vi "MM9.InitDAC.vi"(0 "i ref in":refnum<vi>, 2 "InitObjs":string[](array[string]), 3 "ms timeout (10000)":i32=10000, 5 "error in (no error)":errorcluster) -> (14 "i ref out":refnum<vi>, 16 "InitObjs out":string[](array[string]), 17 "timed out":bool, 19 "error out":errorcluster)   [LabVIEW 2014, in "MM9.lvlib"]
doc: "Initializes the DAC that produces a two stage ramp when triggered."
uses:
  MM9.lvlib
  CS_Core/CSSystem/CoreDefs/CoreDefs.call_type.ctl
  CS_Core/BaseProcess/BaseProcess.descriptor string definition.ctl
  CS_Core/CSSystem/CoreDefs/CoreDefs.rawDataType.ctl
  CS_Core/CSSystem/CoreLib/CoreLib.int 2 byte array.vi
  CS_Core/BaseProcess/BaseProcess.lvlib
  LEBITLib/LEBITLib.lvlib
  CS_Core/CSSystem/CoreLib/CoreLib.lvlib
panel:
  in  "call cluster type":T1={"Object"="", "Selector"="", "CallType"=enum."synchronous", "Async Object"="", "Async Selector"="", "Data Descriptor"="", "Data"=[], "Error #"=0, "Expire"=0}
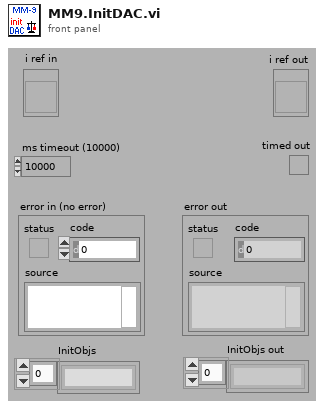
[diagram p1: front panel]
types:
  T1 = typedef "CoreDefs.call_type.ctl" = cluster{"Object":string, "Selector":string, "CallType":enum16{"simple", "synchronous", "asynchronous"}, "Async Object":string, "Async Selector":string, "Data Descriptor":T2, "Data":T3, "Error #":i32, "Expire":u32}
  T2 = typedef "BaseProcess.lvlib/BaseProcess.descriptor string definition.ctl" = string
  T3 = typedef "CoreDefs.rawDataType.ctl" = i8[]
  T4 = typedef "MM9.lvlib/MM9.i attribute.ctl" = cluster{"UsedObjs":string[], "ActScanStep":i32[], "AbortRequest":bool, "StopRequest":bool, "# cycles":i32, "Connected":bool, "MMStatus":T5, "# data":i32, "DIMServices":cluster{"MM6StatusString":string, "MM6StatusID":i32, "discArchiver":string, "discArchiverID":i32, "eventBuilder":string, "eventBuilderID":i32, "GUIIDString":string, "GUIIDStringID":i32}, "dataFile":string, "PGRunning":T6, "ConfigData":T7, "ExtraDataSets":T22}
  T5 = typedef "MM9.lvlib/MM9.status.ctl" = enum16{"loaded", "load_error", "config", "config_error", "init", "init_error", "data_reset", "data_reset_error", "running", "start_error", "run_error", "abort_requested", "aborted", "stop_requested", "stopped", "stop_error", "Connected", "NOTConnected"}
  T6 = typedef "PPG_ABC.lvlib/PPG_ABC.PG_Running.ctl" = i32
  T7 = typedef "LEBITDefs9.lvlib/LEBITDefs.ConfigData.ctl" = cluster{"GenConfig":T8, "Configs":T10[]}
  T8 = typedef "LEBITDefs9.lvlib/LEBITDefs.GenConfig.ctl" = cluster{"Mode":i32, "Logs":T9[]}
  T9 = typedef "LEBITDefs9.lvlib/LEBITDefs.Log.ctl" = cluster{"Name":string, "FctName":string, "Special":string}
  T10 = typedef "LEBITDefs9.lvlib/LEBITDefs.OneConfig.ctl" = cluster{"MCA":T11, "Timing":T12, "Scans":T15[], "FreqDevs":T16[], "CleanDev":T17, "NrCycles":i32, "Specials":T19[], "Delays":T20[], "DAC":T21}
  T11 = typedef "LEBITDefs9.lvlib/LEBITDefs.MCA.ctl" = cluster{"Name":string, "Address":string, "NrChannels":i32, "Gate":i32, "NrPipse":i32, "AcqDelay":i32}
  T12 = typedef "LEBITDefs9.lvlib/LEBITDefs.Timing.ctl" = cluster{"TimeTables":cluster{"TimeTable":T13}[], "Memories":T14[], "ScanX":string, "ScanY":string}
  T13 = typedef "LEBITDefs9.lvlib/LEBITDefs.Timetable.ctl" = dbl[]
  T14 = typedef "LEBITDefs9.lvlib/LEBITDefs.Memory.ctl" = cluster{"Device":string, "ExtTrig":bool, "TT2Use":i32, "PatternTable":string[]}
  T15 = typedef "LEBITDefs9.lvlib/LEBITDefs.ScanDev.ctl" = cluster{"Name":string, "FctName":string, "Values":dbl[], "NrScanVals":i32, "Special":string}
  T16 = typedef "LEBITDefs9.lvlib/LEBITDefs.FreqDev.ctl" = cluster{"Name":string, "Amp":dbl, "CenterFreq":dbl, "Time":dbl}
  T17 = typedef "LEBITDefs9.lvlib/LEBITDefs.CleanDev.ctl" = cluster{"Name":string, "CleanData":T18[]}
  T18 = typedef "LEBITDefs9.lvlib/LEBITDefs.CleanDataType.ctl" = cluster{"Amp":dbl, "Center":dbl, "Plus":dbl, "Minus":dbl, "Time":dbl}
  T19 = typedef "LEBITDefs9.lvlib/LEBITDefs.Special.ctl" = cluster{"Name":string, "FctName":string, "VerySpecial":string, "Data":dbl}
  T20 = typedef "LEBITDefs9.lvlib/LEBITDefs.Delay.ctl" = cluster{"Name":string, "Delay":dbl}
  T21 = typedef "LEBITDefs9.lvlib/LEBITDefs.DAC.ctl" = cluster{"Name":string, "Step1":i32, "Step2":i32}
  T22 = typedef "LEBITDefs9.lvlib/LEBITDefs.ExtraData.ctl" = cluster{"Ions":cluster{"ExcitIonMass":string, "ExcitIonCharge":i32, "CleanIons":cluster{"CleanIonMass":string, "CleanIonCharge":i32}[]}, "TimingDescription":cluster{"TimeTableDescription":cluster{"Times":string[]}[], "PatternTableDescription":cluster{"Pattern":string[]}[]}, "ScanUnits":string[]}[]
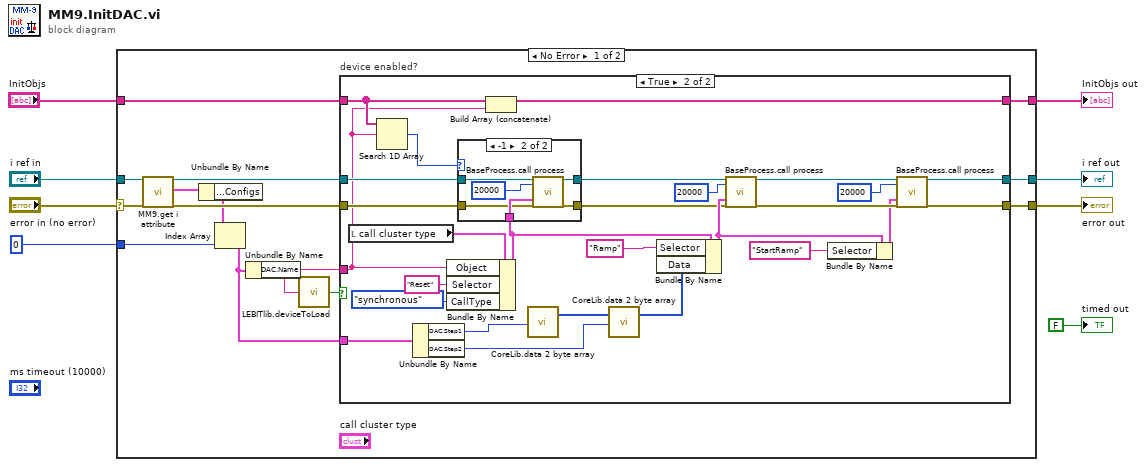
[diagram p0: block diagram]
diagram:
  n1 = case shown="No Error" "error in (no error)" {
    selector: "error in (no error)" -> [w15 w61]
    tunnel: "i ref in" -> [w22 w62]
    tunnel: [w20 w62] -> w7
    tunnel: [w19 w61] -> w6
    tunnel: "InitObjs" -> [w17 w63]
    tunnel: [w16 w63] -> w3
    tunnel: 0 ("index") -> [w9 _]
    frame No Error {
      n2 = call "MM9.get i attribute.vi"("i ref in"=w22, "error in (no error)"=w15) -> ("i ref out"=w21:refnum<vi>, "i attribute"=w11:T4, "error out"=w18:errorcluster)  [unwired: 15 in]
      n3 = Unbundle By Name(w11) -> ("ConfigData.Configs"=w12:T10[])
      n4 = Index Array(array=w12, index=w9) -> (element=w10:T10)
      n5 = Unbundle By Name(w10) -> ("DAC.Name"=w13:string)
      n6 = call "LEBITlib.deviceToLoad.vi"("DeviceName"=w13) -> ("DeviceIsToLoad"=w14:bool)
      n7 = case "device enabled?" shown="True" w14 {
        tunnel: [w25 w31] -> w20
        tunnel: [w24 w30] -> w19
        tunnel: w13 -> [_ w34]
        tunnel: w10 -> [_ w40]
        tunnel: w21 -> [w25 w39]
        tunnel: w18 -> [w24 w38]
        tunnel: w17 -> [w23 w35]
        tunnel: [w23 w33] -> w16
        frame False {
        }
        frame True {
          n8 = local read "call cluster type"() -> (w47:T1)
          n9 = Search 1D Array(1D array=w35, element=w34) -> (index of element=w36:i32)  [unwired: 1 in]
          n10 = Unbundle By Name(w40) -> ("DAC.Step1"=w27:i32, "DAC.Step2"=w26:i32)
          n11 = Bundle By Name(cluster=w47, "Object"=w34, "Selector"="Reset", "CallType"=enum16{"simple", "synchronous", "asynchronous"}."synchronous") -> (w48:T1)
          n12 = case shown="-1" w36 {
            tunnel: [w54 w59] -> w49
            tunnel: w48 -> [_ w58]
            tunnel: w39 -> [w54 w57]
            tunnel: w38 -> [w53 w56]
            tunnel: [w53 w55] -> w37
            frame 0, Default {
            }
            frame -1 {
              n13 = call "BaseProcess.call process.vi"("i ref in"=w57, "timeout (ms)"=20000, "call cluster in"=w58, "error in (no error)"=w56) -> ("i ref out"=w59:refnum<vi>, "error out"=w55:errorcluster)  [unwired: 13 in, 1 out]
            }
          }
          n14 = Build Array (concatenate)(w35, w34) -> (w33:string[])
          n15 = call-poly "CoreLib.data 2 byte array.vi"("i32"=w27) -> ("byteArray out"=w28:T3)  [unwired: 18 in]
          n16 = call-poly "CoreLib.data 2 byte array.vi"("byteArray"=w28, "i32"=w26) -> ("byteArray out"=w29:T3)  [unwired: 17 in]
          n17 = Bundle By Name(cluster=w48, "Selector"="Ramp", "Data"=w29) -> (w44:T1)
          n18 = call "BaseProcess.call process.vi"("i ref in"=w49, "timeout (ms)"=20000, "call cluster in"=w44, "error in (no error)"=w37) -> ("i ref out"=w41:refnum<vi>, "error out"=w42:errorcluster)  [unwired: 13 in, 1 out]
          n19 = Bundle By Name(cluster=w44, "Selector"="StartRamp") -> (w32:T1)
          n20 = call "BaseProcess.call process.vi"("i ref in"=w41, "timeout (ms)"=20000, "call cluster in"=w32, "error in (no error)"=w42) -> ("i ref out"=w31:refnum<vi>, "error out"=w30:errorcluster)  [unwired: 13 in, 1 out]
        }
      }
    }
    frame Error {
    }
  }
  "error out" <- w6
  "i ref out" <- w7
  "InitObjs out" <- w3
  "timed out" <- FALSE ("timed out")
